vi "Teardown.vi"(7 "Queue Actor in":refnum<class "Queue Actor.lvclass">, 11 "Msg State in":refnum<class "Nominal State.lvclass">) -> (5 "Queue Actor out":refnum<class "Queue Actor.lvclass">)   [LabVIEW 2021, in "jettl.lvlib" / "jettl Queue Actor.lvlib" / "Nominal State.lvclass"]
uses:
  Nominal State.lvclass
  Actor/Queue Actor/Queue Actor.lvclass
  Actor/Msgs/Teardown/Teardown Msg/Teardown Msg.lvclass
  C:/git/jettl/src/Actor/Msg/Msg.lvclass
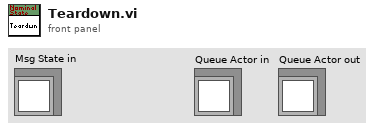
[diagram p1: front panel]
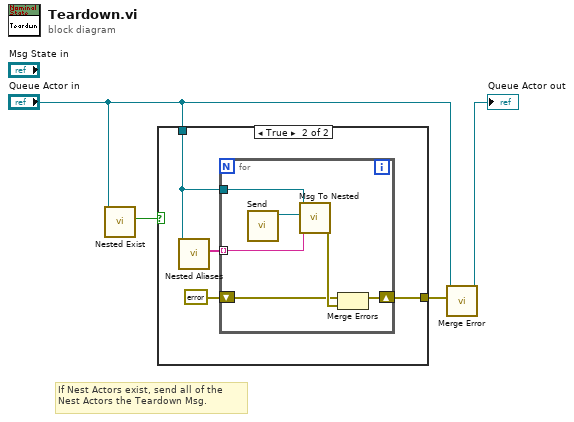
[diagram p0: block diagram]
diagram:
  # "If Nest Actors exist, send all of the Nest Actors the Teardown Msg."
  n1 = call-dynamic "Nested Exist.vi"("Queue Actor in"="Queue Actor in") -> ("Nested Exist?"=w4:bool)  [unwired: 10 in]
  n2 = case shown="True" w4 {
    tunnel: [_ w8] -> w2
    tunnel: "Queue Actor in" -> [_ w6]
    frame False {
    }
    frame True {
      n3 = call-dynamic "Nested Aliases.vi"("Queue Actor in"=w6) -> ("Nested Aliases"=w7:string[])  [unwired: 10 in]
      n4 = for {
        tunnel: w7 -> [w11] mode=indexing
        shift-right: [w14] -> w8
        shift-left: errorcluster {"status"=FALSE, "code"=0, "source"=""} ("error IO") -> [w9]
        tunnel: w6 -> [w13]
        n5 = call "Send.vi"() -> ("Teardown Msg out"=w12:refnum<class "Teardown Msg.lvclass">)  [unwired: 11 in]
        n6 = call-dynamic "Msg To Nested.vi"("Alias"=w11, "Msg"=w12, "Queue Actor in"=w13) -> ("error out"=w10:errorcluster)  [unwired: 8 in]
        n7 = Merge Errors(w9, w10) -> (w14:errorcluster)
      }
    }
  }
  n8 = call-dynamic "Merge Error.vi"("Error"=w2, "Set Error in"="Queue Actor in") -> ("Set Error out"=→"Queue Actor out":refnum<class "Queue Actor.lvclass">)  [unwired: 9 in]
